vi "AddChildren.vi"(8 "error in (no error)":errorcluster, 9 "Enqueuer":refnum<class "Message Enqueuer.lvclass">, 10 "Actor Name":string, 11 "TopLevel in":refnum<class "TopLevel.lvclass">) -> (0 "error out":errorcluster, 3 "TopLevel out":refnum<class "TopLevel.lvclass">)   [LabVIEW 2019, in "TopLevel.lvlib" / "TopLevel.lvclass"]
uses:
  TopLevel.lvclass
  <vilib>/ActorFramework/Message Enqueuer/Message Enqueuer.lvclass
  TopLevel.lvclass/TopLevel.ctl
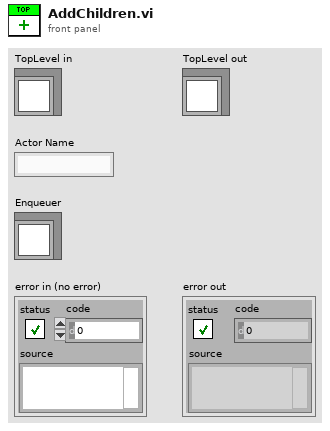
[diagram p1: front panel]
types:
  T1 = map{string, refnum<class "Message Enqueuer.lvclass">}
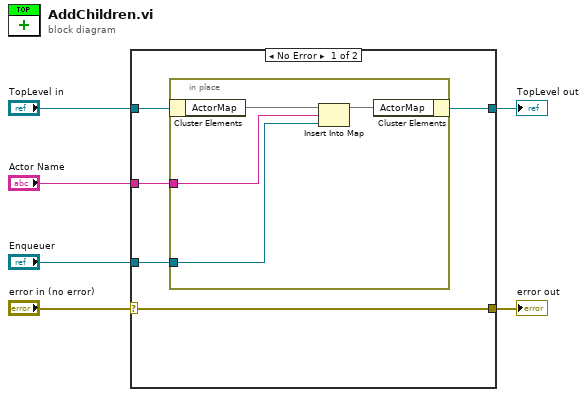
[diagram p0: block diagram]
diagram:
  n1 = case shown="No Error" "error in (no error)" {
    selector: "error in (no error)" -> [w7 w17]
    tunnel: [w7 w17] -> w5
    tunnel: [w8 w16] -> w3
    tunnel: "TopLevel in" -> [w11 w16]
    tunnel: "Actor Name" -> [w10 _]
    tunnel: "Enqueuer" -> [w9 _]
    frame No Error {
      n2 = in-place {
        in-place-border: w10 -> [w13]
        in-place-border: w9 -> [w12]
        n3 = in-place-cluster #1(w11) -> ("ActorMap"=w15:T1)
        n4 = Insert Into Map(map in=w15, key=w13, value=w12) -> (map out=w14:T1)  [unwired: 2 out]
        n5 = in-place-cluster #1("ActorMap"=w14) -> (w8:refnum<class "TopLevel.lvclass">)
      }
    }
    frame Error {
    }
  }
  "error out" <- w5
  "TopLevel out" <- w3
